vi "getPath.vi"(8 "error in (no error)":errorcluster, 11 "FileReader in":refnum<class "FileReader.lvclass">) -> (0 "error out":errorcluster, 2 "Path":path=path "C:/Users/Administrator/Desktop/Crete/Data/2014/1411/141126/Scripts/Instrument Scripts/Dio64.csv", 3 "FileReader out":refnum<class "FileReader.lvclass">)   [LabVIEW 2011, in "Tools.lvlib" / "Filing.lvlib" / "FileReader.lvclass"]
uses:
  FileReader.lvclass
  FileReader.lvclass/FileReader.ctl
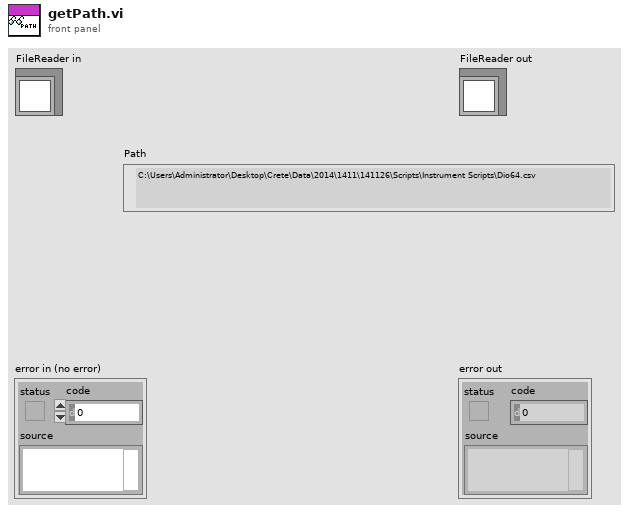
[diagram p1: front panel]
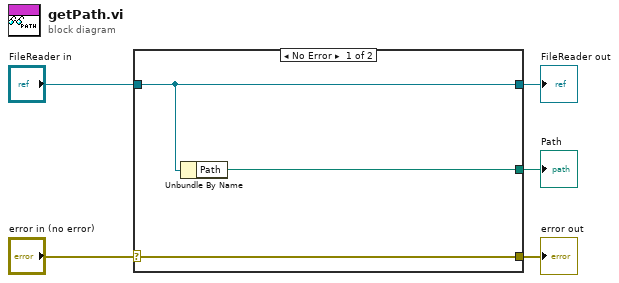
[diagram p0: block diagram]
diagram:
  n1 = case shown="No Error" "error in (no error)" {
    selector: "error in (no error)" -> [w8 w9]
    tunnel: [w8 w9] -> w4
    tunnel: [w7 w10] -> w2
    tunnel: "FileReader in" -> [w7 w10]
    tunnel: [w6 _] -> w1
    frame No Error {
      n2 = Unbundle By Name(w7) -> ("Path"=w6:path)
    }
    frame Error {
    }
  }
  "error out" <- w4
  "FileReader out" <- w2
  "Path" <- w1
